vi "Exercise1.1.vi"() -> ()   [LabVIEW 2019]
panel:
  out "Last Random Number":dbl
  out "Waveform Chart":dbl(graph)
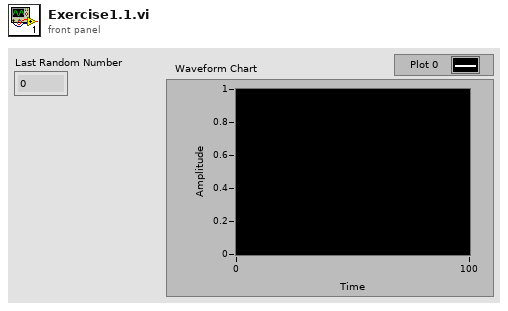
[diagram p1: front panel]
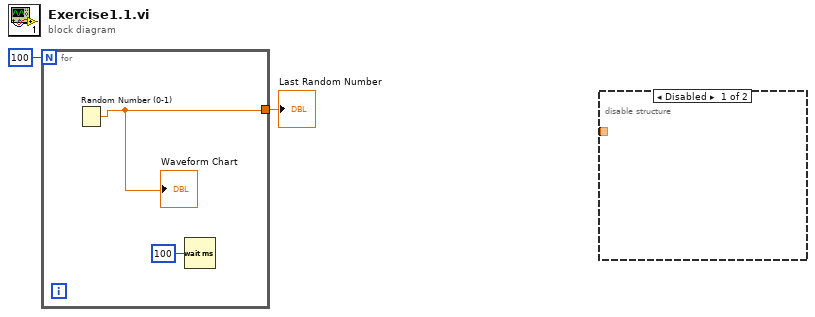
[diagram p0: block diagram]
diagram:
  n1 = for {
    N: 100 -> [_]
    tunnel: [w3] -> w1
    n2 = Random Number (0-1)() -> (number: 0 to 1=w3:dbl)
    "Waveform Chart" <- w3
    n3 = Wait (ms)(milliseconds to wait=u32 100) -> ()  [unwired: 1 out]
  }
  "Last Random Number" <- w1
  n4 = disable-structure shown="Disabled" {
    disable-tunnel: _ -> [w5 _]
    frame Disabled {
    }
    frame Enabled {
    }
  }
